vi "Subject Controller_Create.vi"(8 "error in (no error)":errorcluster, 11 "reference in":refnum<class "Subject Controller.lvclass">) -> (0 "error out":errorcluster, 3 "reference out":refnum<class "Subject Controller.lvclass">)   [LabVIEW 2015, in "Subject Controller.lvclass"]
doc: "Constructor."
uses:
  Subject Controller.lvclass
  <vilib>/addons/_AddQ/G#Object/utils/G#Object_CreateMethod.ctl
  <vilib>/addons/_AddQ/G#Object/G#Object.lvclass
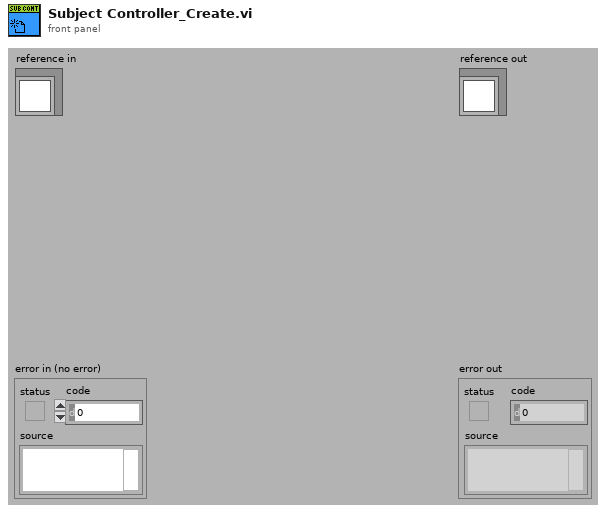
[diagram p1: front panel]
types:
  T1 = typedef "G#Object.lvclass/G#Object_CreateMethod.ctl" = enum16{"Create", "Create or look up existing", "Look up existing"}
  T2 = typedef "Subject Controller.lvclass/ClassAttributesRef.ctl" = refnum<data-value>
  T3 = typedef "Subject Controller.lvclass/ClassAttributes.ctl" = cluster{"Dummy":bool, "subject_controller_ref":refnum<class "Subject Controller.lvclass">}
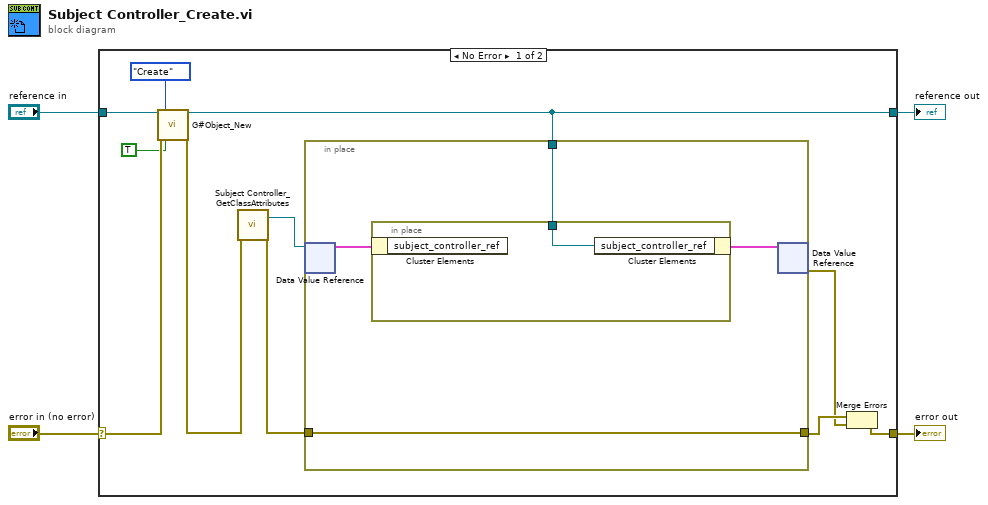
[diagram p0: block diagram]
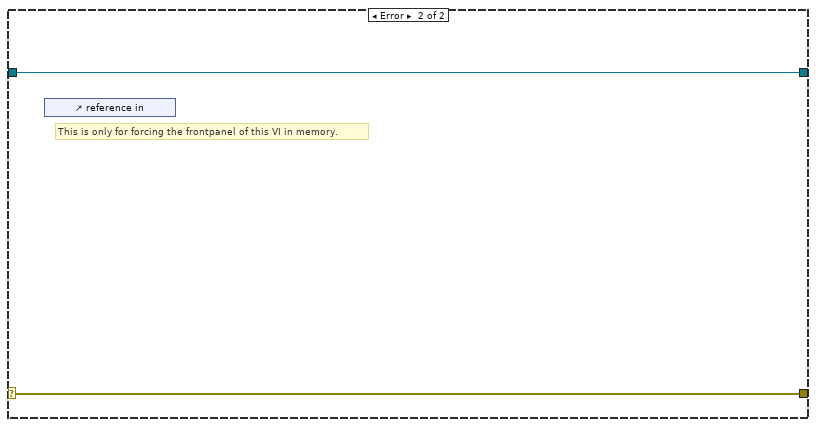
[diagram p2: hidden frame]
diagram:
  n1 = case shown="No Error" "error in (no error)" {
    selector: "error in (no error)" -> [w14 w22]
    tunnel: [w13 w22] -> w3
    tunnel: [w8 w21] -> w1
    tunnel: "reference in" -> [w15 w21]
    frame No Error {
      n2 = call <vilib>:"G#Object_New.vi"("reference in"=w15, "error in (no error)"=w14, "create method"=G#Object_CreateMethod."Create", "user counter (T)?"=TRUE ("User Counter")) -> ("reference out"=w8:refnum<class "Subject Controller.lvclass">, "error out"=w7:errorcluster)  [unwired: 13 in, 1 out]
      n3 = call "Subject Controller_GetClassAttributes.vi"("error in (no error)"=w7) -> ("class attributes ref"=w9:T2, "error out"=w6:errorcluster)  [unwired: 15 in, 2 out]
      n4 = in-place {
        in-place-border: w6 -> [w17]
        in-place-border: [w17] -> w11
        in-place-border: w8 -> [w16]
        n5 = in-place-dvr #1(w9) -> (w18:T3)  [unwired: 1 out]
        n6 = in-place {
          in-place-border: w16 -> [w20]
          n7 = in-place-cluster #2(w18) -> ()  [unwired: 1 out]
          n8 = in-place-cluster #2("subject_controller_ref"=w20) -> (w19:T3)
        }
        n9 = in-place-dvr #1(w19) -> (w10:errorcluster)  [unwired: 1 out]
      }
      n10 = Merge Errors(w11, w10) -> (w13:errorcluster)
    }
    frame Error {
      # "This is only for forcing the frontpanel of this VI in memory."
      n11 = control-ref of="reference in"() -> ()  [unwired: 1 out]
    }
  }
  "error out" <- w3
  "reference out" <- w1
